vi "Refresh Rooms Status.vi"(0 "File Data Manager in":refnum<class "File Data Manager.lvclass">, 11 "error in (no error)":errorcluster) -> (4 "File Data Manager out":refnum<class "File Data Manager.lvclass">, 15 "error out":errorcluster)   [LabVIEW 2023, in "File Data Manager.lvlib" / "File Data Manager.lvclass"]
uses:
  File Data Manager.lvclass
  File Data Manager.lvclass/File Data Manager.ctl
  <vilib>/ActorFramework/Actor/Actor.lvclass
  Interfaces/Incoming Hotel Management Tool Model Interface Messages/Refresh Rooms Status Msg/Refresh Rooms Status Msg.lvclass
  C:/Users/bhaghyaraj/Trainings/NI Actor Frameowork/SDLC/Central Data Manager/Central Data Manager/Central Data Manager.lvclass
  C:/Users/bhaghyaraj/Trainings/NI Actor Frameowork/SDLC/Model Base/Model Base/Model Base.lvclass
  C:/Program Files/National Instruments/LabVIEW 2023/vi.lib/ActorFramework/Actor/Actor.lvclass
  C:/Users/bhaghyaraj/Trainings/NI Actor Frameowork/SDLC/Interfaces/Model Base/Incoming Model Base Interface.lvclass
  C:/Users/bhaghyaraj/Trainings/NI Actor Frameowork/SDLC/File Data Manager/File Data Manager/File Data Manager.lvclass
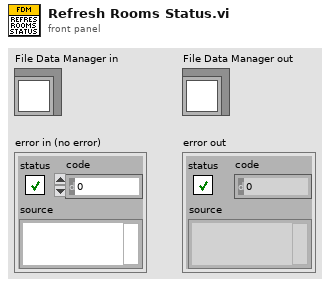
[diagram p1: front panel]
types:
  T1 = typedef "Central Data Manager.lvlib/Central Data Manager.lvclass/Room Size Details.ctl" = cluster{"Size":string, "Cost Per Day (Rs)":u32, "Occupancy Limit (Adult)":u32, "Occupancy Limit (Children)":u32}
  T2 = typedef "Central Data Manager.lvlib/Central Data Manager.lvclass/Room Details.ctl" = cluster{"Room No":string, "Room Size":string, "Room Occupancy Status":T3, "Guest Details":T4, "Occupancy Count (Adult)":u32, "Occupancy Count (Children)":u32, "Check-in Time":timestamp, "Check-out Time":timestamp}
  T3 = typedef "Central Data Manager.lvlib/Central Data Manager.lvclass/Room Occupancy Status.ctl" = enum16{"Not Occupied", "Occupied", "Under Maintainance", "Not Servicable"}
  T4 = typedef "Central Data Manager.lvlib/Central Data Manager.lvclass/Guest Details.ctl" = cluster{"Contact Number":string, "Primary Guest Name":string}
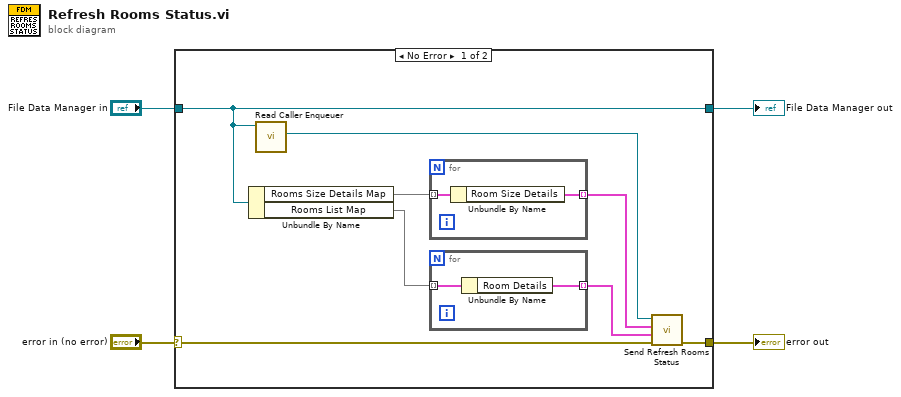
[diagram p0: block diagram]
diagram:
  n1 = case shown="No Error" "error in (no error)" {
    selector: "error in (no error)" -> [w9 w18]
    tunnel: [w8 w18] -> w3
    tunnel: [w7 w17] -> w1
    tunnel: "File Data Manager in" -> [w7 w17]
    frame No Error {
      n2 = Unbundle By Name(w7) -> ("Rooms Size Details Map"=w5:map{string, T1}, "Rooms List Map"=w6:map{string, T2})
      n3 = call <vilib>:"Read Caller Enqueuer.vi"("Actor"=w7) -> ("Caller Enqueuer"=w12:refnum<class "Message Enqueuer.lvclass">)  [unwired: 10 in]
      n4 = for {
        tunnel: [w15] -> w11 mode=indexing
        tunnel: w5 -> [w16] mode=indexing
        n5 = Unbundle By Name(w16) -> ("Room Size Details"=w15:T1)
      }
      n6 = for {
        tunnel: [w13] -> w10 mode=indexing
        tunnel: w6 -> [w14] mode=indexing
        n7 = Unbundle By Name(w14) -> ("Room Details"=w13:T2)
      }
      n8 = call "Send Refresh Rooms Status.vi"("error in (no error)"=w9, "Rooms List"=w10, "Room Size Details"=w11, "Message Enqueuer"=w12) -> ("error out"=w8:errorcluster)  [unwired: 6 in, 1 out]
    }
    frame Error {
    }
  }
  "error out" <- w3
  "File Data Manager out" <- w1
